vi "弯曲验证.vi"(0 "文件路径输入控件":path) -> (1 "XY图":cluster{"Y":dbl[], "Y":dbl[]}[](graph), 2 "弯曲刚度值":dbl)   [LabVIEW 2016]
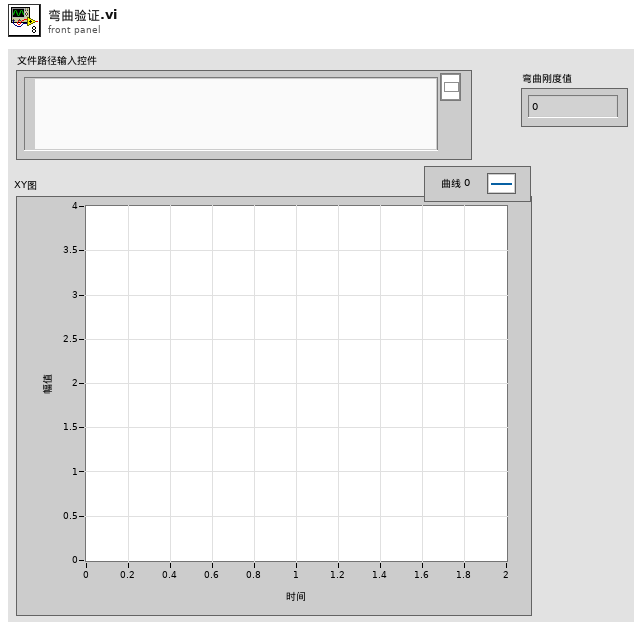
[diagram p1: front panel]
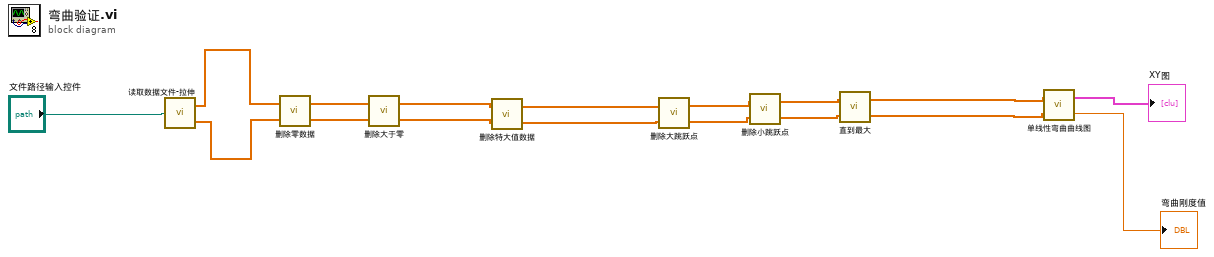
[diagram p0: block diagram]
diagram:
  n1 = call "读取数据文件-拉伸.vi"("文件路径（使用对话框）"="文件路径输入控件") -> ("第一列"=w16:dbl[], "第二列"=w15:dbl[])
  n2 = call "删除零数据.vi"("数组－数值 2"=w15, "数组－数值"=w16) -> ("第二列"=w13:dbl[], "第一列"=w14:dbl[])
  n3 = call "删除大于零.vi"("数组－数值 2"=w13, "数组－数值"=w14) -> ("第二列"=w3:dbl[], "第一列"=w4:dbl[])
  n4 = call "删除特大值数据.vi"("数组－数值 2"=w3, "数组－数值"=w4) -> ("数组 6"=w1:dbl[], "数组 5"=w2:dbl[])
  n5 = call "删除大跳跃点.vi"("数组－数值 2"=w1, "数组－数值"=w2) -> ("数组 6"=w11:dbl[], "数组 5"=w12:dbl[])
  n6 = call "删除小跳跃点.vi"("数组－数值 2"=w11, "数组－数值"=w12) -> ("第二列"=w9:dbl[], "第一列"=w10:dbl[])
  n7 = call "直到最大.vi"("数组－数值 2"=w9, "数组－数值"=w10) -> ("子数组 2"=w5:dbl[], "子数组"=w6:dbl[])
  n8 = call "单线性弯曲曲线图.vi"("数组－数值 2"=w5, "数组－数值"=w6) -> ("弯曲刚度值"=→"弯曲刚度值":dbl, "XY Graph"=→"XY图":cluster{"Y":dbl[], "Y":dbl[]}[])
